vi "JenkinsUnitTests.vi"(11 "Args":string[](array[string])) -> (2 "Output":string, 3 "Exit Code":i32)   [LabVIEW 2018]
uses:
  <vilib>/addons/_JKI Toolkits/Caraya/classes/Test Suite/Define Test Suite (JUnit Report).vi
  <vilib>/addons/_JKI Toolkits/Caraya/classes/Test Suite/Test Suite.lvclass
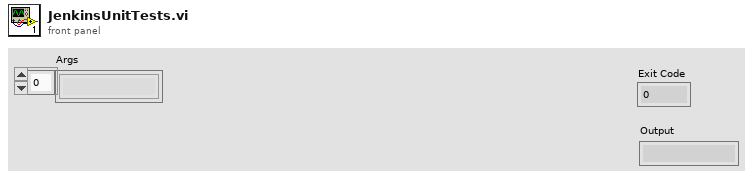
[diagram p1: front panel]
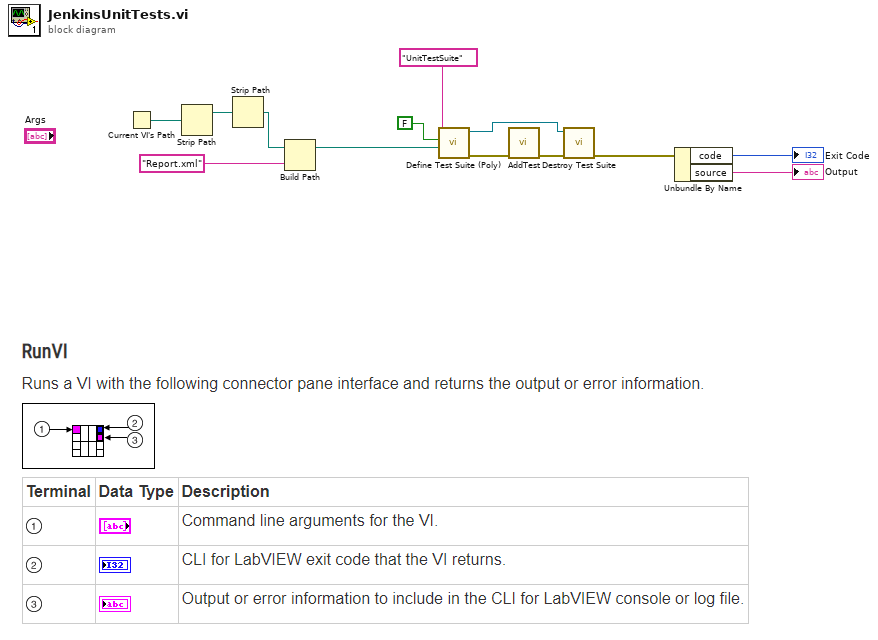
[diagram p0: block diagram]
diagram:
  n1 = Current VI's Path() -> (path=w6:path)
  n2 = Strip Path(path=w6) -> (stripped path=w5:path)  [unwired: 1 out]
  n3 = Strip Path(path=w5) -> (stripped path=w4:path)  [unwired: 1 out]
  n4 = Build Path(base path=w4, name or relative path="Report.xml" ("Report Path")) -> (appended path=w8:path)
  n5 = call-poly <vilib>:"Define Test Suite (Poly).vi"("Report Path"=w8, "Interactive"=FALSE, "Label (VI Title)"="UnitTestSuite") -> ("error out"=w3:errorcluster, "Test Suite"=w2:refnum<class "Test Suite.lvclass">)  [unwired: 7 in]
  n6 = call "AddTest.vi"("error in (no error)"=w3) -> ("error out"=w1:errorcluster)  [unwired: 10 in]
  n7 = call-dynamic "Destroy Test Suite.vi"("error in (no error)"=w1, "Test Suite in"=w2) -> ("error out"=w11:errorcluster)  [unwired: 9 in]
  n8 = Unbundle By Name(w11) -> ("code"=→"Exit Code":i32, "source"=→"Output":string)
